vi "SpawnProgram.vi"(6 "Control Name":string="Robot REPL", 8 "Code Ref":refnum<vi>, 10 "Data In":T1={"Port"="", "All Code"="Hi"}, 11 "Dialog":enum16{"REPL", "Help"}(ring)) -> ()   [LabVIEW 2019]
uses:
  <userlib>/MicroPython/VIs/uPythonX/PythonData.ctl
  <userlib>/MicroPython/VIs/uPythonX/uPythonX.xctl
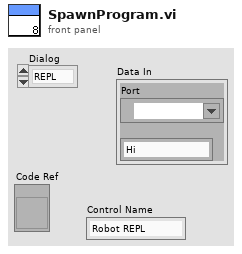
[diagram p1: front panel]
types:
  T1 = typedef "uPythonX.xctl/PythonData.ctl" = cluster{"Port":refnum<visa-resource-name>, "All Code":string}
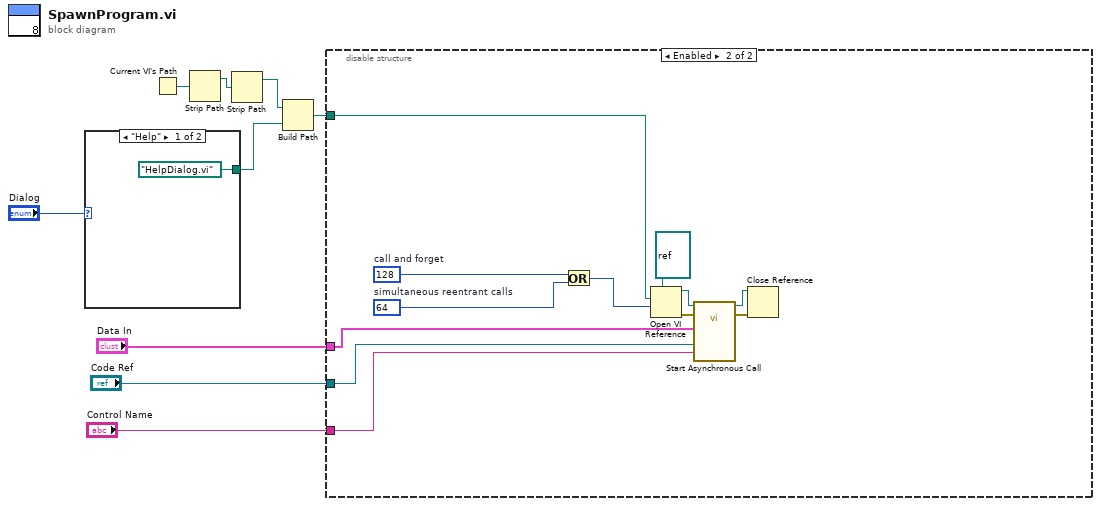
[diagram p0: block diagram]
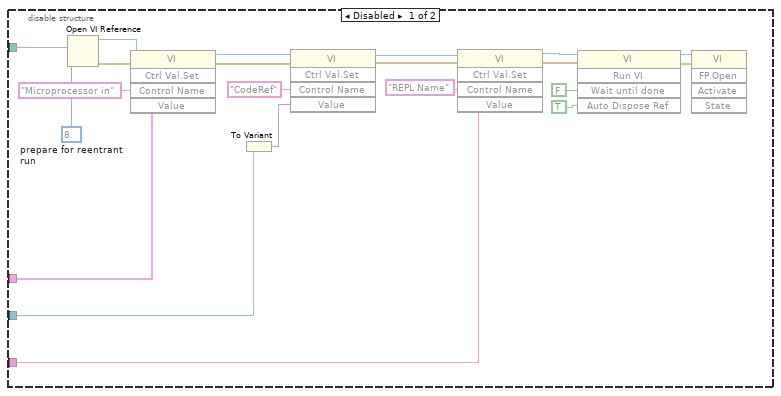
[diagram p2: hidden frame]
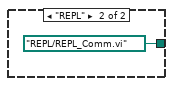
[diagram p3: hidden frame]
diagram:
  n1 = case shown="\"Help\"" "Dialog" {
    tunnel: [path "HelpDialog.vi" ("Name") path "REPL/REPL_Comm.vi" ("Name")] -> w5
    frame "Help" {
    }
    frame "REPL" {
    }
  }
  n2 = Current VI's Path() -> (path=w6:path)
  n3 = Strip Path(path=w6) -> (stripped path=w7:path)  [unwired: 1 out]
  n4 = Strip Path(path=w7) -> (stripped path=w8:path)  [unwired: 1 out]
  n5 = Build Path(base path=w8, name or relative path=w5) -> (appended path=w9:path)
  n6 = disable-structure shown="Enabled" {
    disable-tunnel: w9 -> [w30 w36]
    disable-tunnel: "Data In" -> [w27 w33]
    disable-tunnel: "Code Ref" -> [w20 w35]
    disable-tunnel: "Control Name" -> [w13 w34]
    frame Disabled {
      w12 = 8  # prepare for reentrant run
      n7 = Open VI Reference(vi path=w30, options=w12) -> (vi reference=w25:refnum<vi>, error out=w24:errorcluster)  [unwired: 4 in]
      n8 = invoke class="VI" method="Ctrl Val.Set"(reference=w25, error in=w24, "Control Name"="Microprocessor in", "Value"=w27) -> (reference out=w23:refnum<vi>, error out=w22:errorcluster)  [unwired: 1 in, 3 out]
      n9 = To Variant(anything=w20) -> (Variant=w19:variant)
      n10 = invoke class="VI" method="Ctrl Val.Set"(reference=w23, error in=w22, "Control Name"="CodeRef", "Value"=w19) -> (reference out=w17:refnum<vi>, error out=w15:errorcluster)  [unwired: 1 in, 3 out]
      n11 = invoke class="VI" method="Ctrl Val.Set"(reference=w17, error in=w15, "Control Name"="REPL Name", "Value"=w13) -> (reference out=w16:refnum<vi>, error out=w14:errorcluster)  [unwired: 1 in, 3 out]
      n12 = invoke class="VI" method="Run VI"(reference=w16, error in=w14, "Wait until done"=FALSE ("Wait Until Done"), "Auto Dispose Ref"=TRUE ("Auto Dispose Reference")) -> (reference out=w31:refnum<vi>, error out=w32:errorcluster)  [unwired: 1 in, 3 out]
      n13 = invoke class="VI" method="FP.Open"(reference=w31, error in=w32) -> ()  [unwired: 3 in, 5 out]
    }
    frame Enabled {
      w43 = 64  # simultaneous reentrant calls
      w44 = 128  # call and forget
      n14 = Or(x=w44, y=w43) -> (x .or. y?=w40:i32)
      n15 = Open VI Reference(type specifier VI Refnum (for type only)=refnum<vi> refnum ("reference"), vi path=w36, options=w40) -> (vi reference=w41:refnum<vi>, error out=w42:errorcluster)  [unwired: 3 in]
      n16 = call-by-ref "Start Asynchronous Call"(reference=w41, error in=w42, "REPL Name"=w34, "CodeRef"=w35, "Microprocessor in"=w33) -> (reference out=w37:refnum<vi>, error out=w38:errorcluster)  [unwired: 8 in, 1 out]
      n17 = Close Reference(reference=w37, error in (no error)=w38) -> ()  [unwired: 1 out]
    }
  }
